vi "hplc_analyze.vi"(10 "File Path":string="\\\\KINETIX-1\\Chem32\\1\\DATA\\KCA_HWE\\\n\\\\KINETIX-1\\Chem32\\1\\DATA\\KCA_HWE") -> (0 "error out":errorcluster)   [LabVIEW 2015]
panel:
  # "HPLC Analysis"
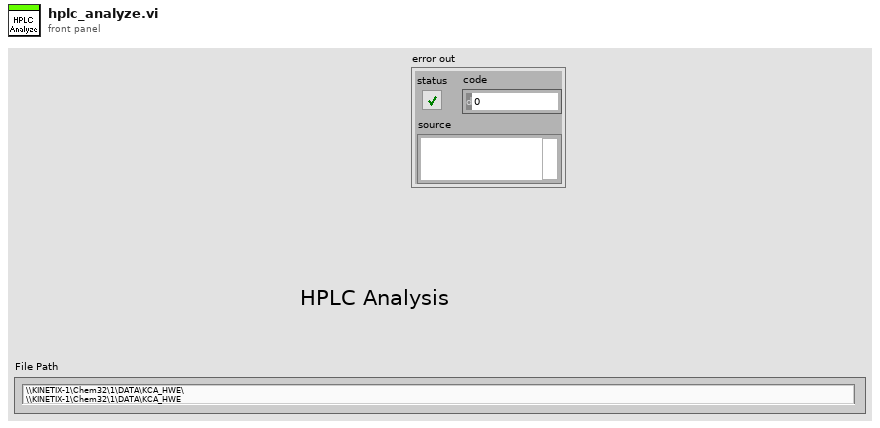
[diagram p1: front panel]
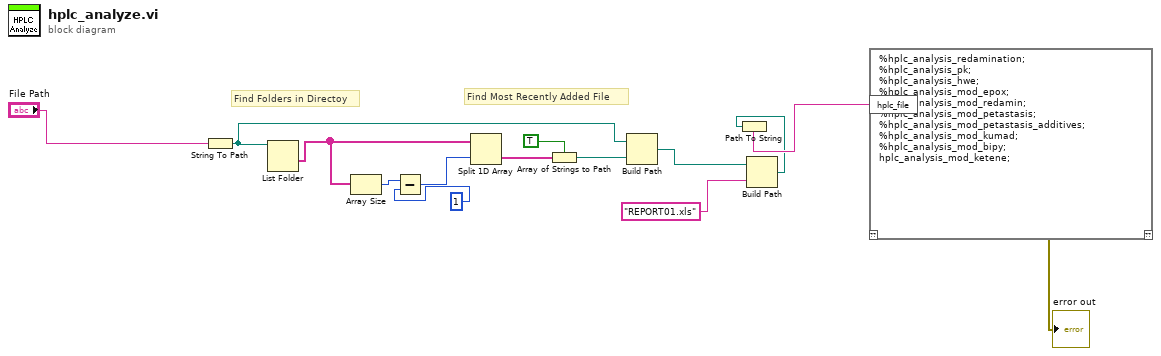
[diagram p0: block diagram]
diagram:
  # "Find Most Recently Added File"
  # "Find Folders in Directoy"
  n1 = String To Path(string="File Path") -> (path=w11:path)
  n2 = List Folder(path=w11) -> (folder names=w9:string[])  [unwired: 3 in, 3 out]
  n3 = Array Size(array=w9) -> (size(s)=w8:i32)
  n4 = Subtract(x=w8, y=1 ("index")) -> (x-y=w6:i32)
  n5 = Split 1D Array(array=w9, index=w6) -> (second subarray=w14:string[])  [unwired: 1 out]
  n6 = Array of Strings to Path(0:w14, 1:TRUE ("relative")) -> (2:w12:path)
  n7 = Build Path(base path=w11, name or relative path=w12) -> (appended path=w4:path)
  n8 = Build Path(base path=w4, name or relative path="REPORT01.xls") -> (appended path=w2:path)
  n9 = Path To String(path=w2) -> (string=w5:string)
  n10 = script code="%hplc_analysis_redamination;\n%hplc_analysis_pk;\n%hplc_analysis_hwe;\n%hplc_analysis_mod_epox;\n%hplc_analysis_mod_redamin;\n%hplc_analysis_mod_petastasis;\n%hplc_analysis_mod_petastasis_additives;\n%hplc_analysis_mod_kumad;\n%hplc_analysis_mod_bipy;\nhplc_analysis_mod_ketene;"("hplc_file"=w5) -> ("??"=→"error out":errorcluster)  [unwired: 1 in]
